vi "VAJ conti move.vi"(7 "move?":bool, 8 "error in (no error)":errorcluster, 9 "Position in":T1, 11 "move in":T3[](array[typedef])) -> (0 "error out":errorcluster, 1 "Position out":T1, 4 "Position out 2":T1)   [LabVIEW 2019]
uses:
  move cluster(VAJ).ctl
  move/position cluster.ctl
  <vilib>/Platform/TimedLoop/XDataNode/timing_clust.ctl
  <vilib>/Platform/TimedLoop/XDataNode/nitl_modes.ctl
  <vilib>/Platform/TimedLoop/XDataNode/wakeup.ctl
  <vilib>/platform/TimedLoop/XDataNode/XDataNode.xnode
  <vilib>/Platform/TimedLoop/XDataNode/XDNodeRunTimeDep.lvlib
panel:
  out "encoder array":dbl[](array[numeric])
  out "Waveform Chart":T2(graph)
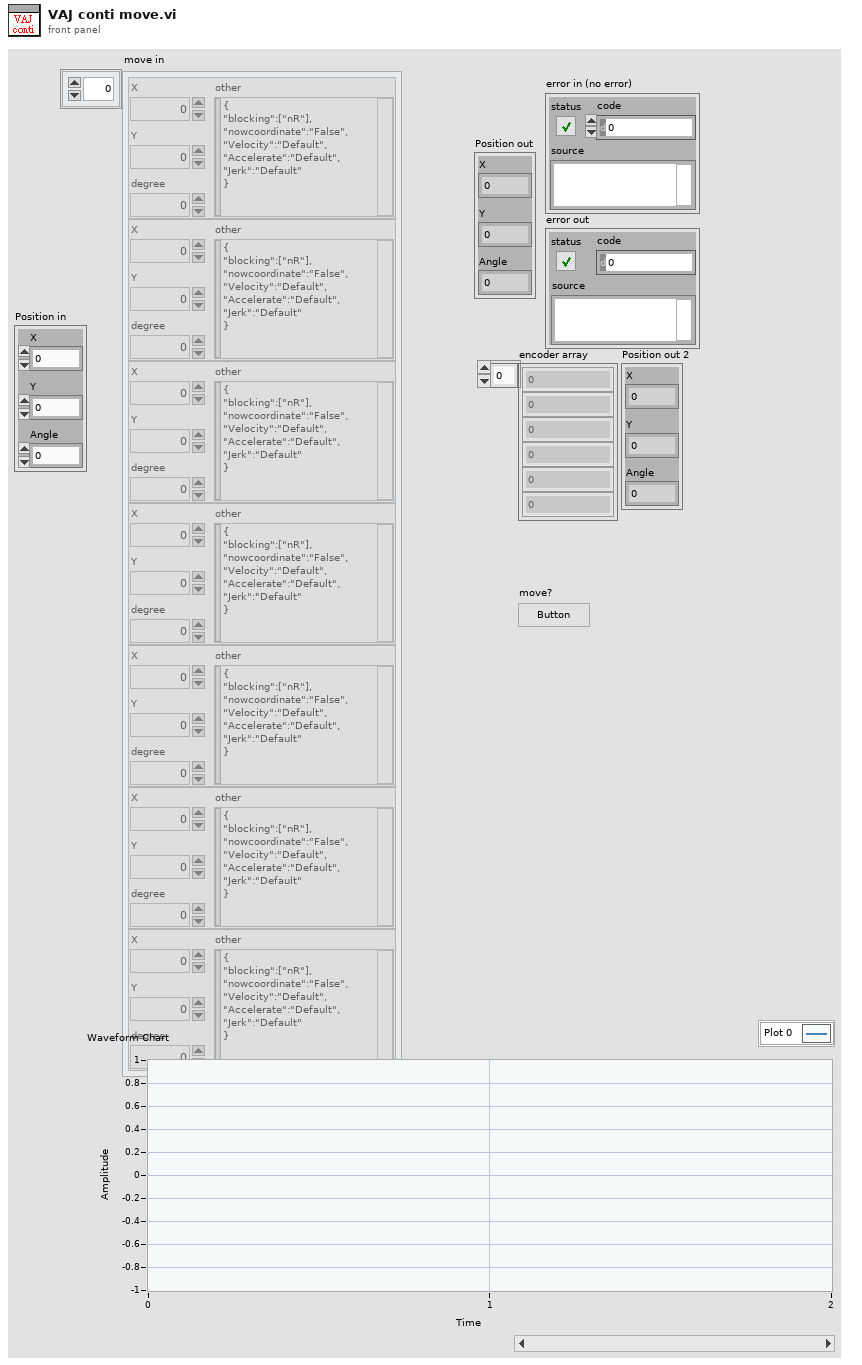
[diagram p1: front panel]
types:
  T1 = typedef "position cluster.ctl" = cluster{"X":dbl, "Y":dbl, "Angle":dbl}
  T2 = cluster{"[0]":dbl, "[1]":dbl, "[2]":dbl, "[3]":dbl, "[4]":dbl, "[5]":dbl, "[6]":dbl, "[7]":dbl, "[8]":dbl}
  T3 = typedef "move cluster(VAJ).ctl" = cluster{"X":dbl, "Y":dbl, "degree":dbl, "other":string}
  T4 = cluster{"Array":cluster{"Numeric":dbl, "Numeric":dbl}[], "direction out":dbl[], "rotate?":bool}[]
  T5 = typedef "BNO055 gyro 3axis.ctl" = cluster{"yaw":dbl, "pitch":dbl, "roll":dbl}
  T6 = typedef "XDNodeRunTimeDep.lvlib/timing_clust.ctl" = cluster{"Expected End [f-1]":u64, "Actual End [f-1]":u64, "Finished Late? [f-1]":bool, "Expected End [i-1]":u64, "Actual End [i-1]":u64, "Finished Late? [i-1]":bool, "Expected Start [i]":u64, "Actual Start [i]":u64, "Expected Start [f]":u64, "Actual Start [f]":u64, "Source Name":string, "Structure Name":string, "Period":i64, "Deadline":i64, "Offset":i64, "Start":i64, "Priority":i32, "Timeout":i32, "Mode":T7, "Wakeup Reason":T8, "Error":errorcluster, "Source Type":string, "Secondary Source Type":string, "Global End Time":u64, "Global Start Time":u64, "Frame Duration":u64, "Iteration Duration":u64, "Assigned CPU":i32, "I/O Scan Engine Mode":u32}
  T7 = typedef "XDNodeRunTimeDep.lvlib/nitl_modes.ctl" = enum32{"No Change", "Process missed periods, maintain original phase", "Discard missed periods, maintain original phase", "Process missed periods, ignore original phase", "Discard missed periods, ignore original phase"}
  T8 = typedef "XDNodeRunTimeDep.lvlib/wakeup.ctl" = enum32{"Normal", "Aborted", "Asynchronous wakeup", "Timing source error", "Timed loop error", "Timeout"}
  T9 = cluster{"Array":cluster{"Numeric":dbl, "Numeric":dbl}[], "direction out":dbl[], "rotate?":bool}
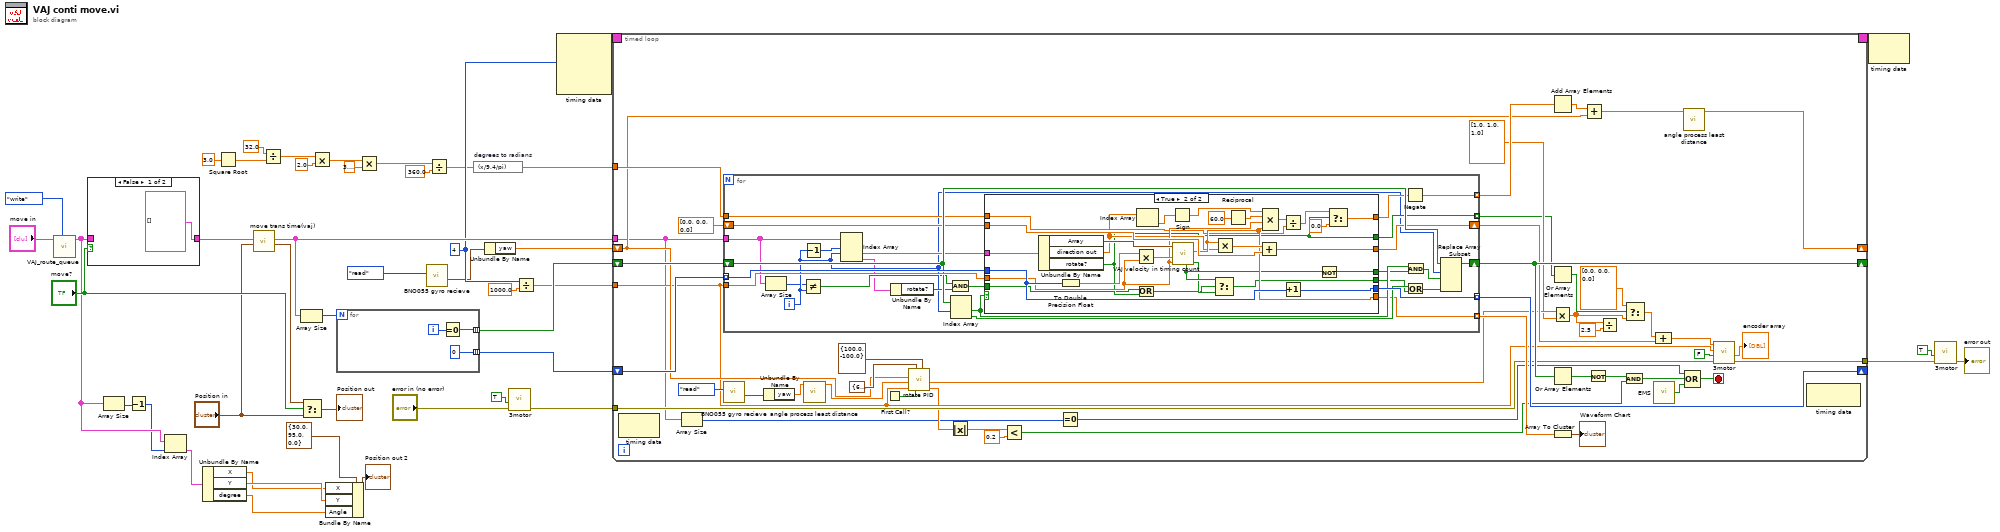
[diagram p0: block diagram]
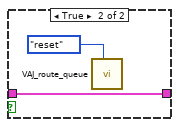
[diagram p2: hidden frame]
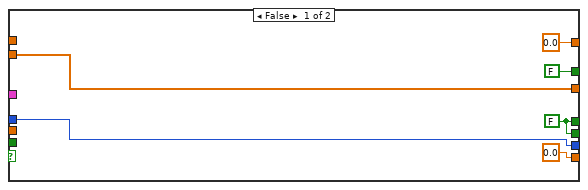
[diagram p3: hidden frame]
diagram:
  w39 = i64 4 ("Period")
  n1 = call "VAJ_route_queue.vi"("set"=enum16{"reset", "write"}."write", "move in"="move in") -> ("s? t:f"=w8:T3[])  [unwired: 9 in]
  n2 = case shown="False" "move?" {
    tunnel: [T3[] [] ("s? t:f") w48] -> w14
    tunnel: w8 -> [_ w48]
    frame False {
    }
    frame True {
      n3 = call "VAJ_route_queue.vi"("set"=enum16{"reset", "write"}."reset") -> ()  [unwired: 10 in, 1 out]
    }
  }
  n4 = Array Size(array=w8) -> (size(s)=w9:i32)
  n5 = Decrement(x=w9) -> (x-1=w7:i32)
  n6 = Index Array(array=w8, index=w7) -> (element=w6:T3)
  n7 = Unbundle By Name(w6) -> ("X"=w1:dbl, "Y"=w2:dbl, "degree"=w3:dbl)
  n8 = Square Root(x=3.0) -> (sqrt(x)=w23:dbl)
  n9 = call "move trans time(vaj)"("Position in"="Position in", "move in"=w14) -> ("Position out"=w11:T1, "speed create"=w43:T4)  [unwired: 8 in]
  n10 = Divide(x=32.0, y=w23) -> (x/y=w25:dbl)
  n11 = Array Size(array=w43) -> (size(s)=w42:i32)
  n12 = Select(t=w11, s="move?", f="Position in") -> (s? t:f=→"Position out":T1)
  n13 = Multiply(x=w25, y=2.0) -> (x*y=w28:dbl)
  n14 = Bundle By Name(cluster=T1 {"X"=30.0, "Y"=95.0, "Angle"=0.0} ("Position out 2"), "X"=w1, "Y"=w2, "Angle"=w3) -> (→"Position out 2":T1)
  n15 = for {
    N: w42 -> [_]
    tunnel: [w50] -> w41 mode=indexing
    tunnel: [0] -> w40 mode=indexing
    i -> [w49]
    n16 = Equal To 0?(x=w49) -> (x = 0?=w50:bool)
  }
  n17 = Multiply(x=w28, y=3.141592653589793) -> (x*y=w29:dbl)
  n18 = call "BNO055 gyro recieve.vi"("Enum"=enum16{"read", "write"}."read") -> ("read"=w20:T5)  [unwired: 10 in]
  n19 = Divide(x=w29, y=360.0) -> (x/y=w18:dbl)
  n20 = expression code="(x/9.4/pi)" "degrees to radians"(w18) -> (w17:dbl)
  n21 = Unbundle By Name(w20) -> ("yaw"=w19:dbl)
  n22 = call "3motor.vi"("error in (no error)"="error in (no error)", "Reset"=TRUE) -> ("error out"=w36:errorcluster)  [unwired: 8 in, 1 out]
  n23 = Divide(x=w39, y=1000.0) -> (x/y=w37:dbl)
  n24 = node-c288(w39) -> (w45:T6)  [unwired: 3 in]
  n25 = timed-loop {
    timing: w45 -> [_]
    timing-out: [_] -> w44
    tunnel: w43 -> [w59]
    shift-right: [w94] -> _
    shift-left: w41 -> [w98]
    shift-right: [w96] -> _
    shift-left: w40 -> [w97]
    tunnel: w37 -> [w73]
    tunnel: w36 -> [w87]
    tunnel: [w86] -> w32
    tunnel: w17 -> [w82]
    shift-right: [w79] -> _
    shift-left: w19 -> [w74]
    stop <- w85 stop-if-true
    n26 = node-c288() -> ()  [unwired: 1 in, 1 out]
    n27 = Array Size(array=w59) -> (size(s)=w58:i32)
    n28 = for {
      tunnel: w59 -> [w99]
      tunnel: w97 -> [w125] mode=indexing
      tunnel: [w124] -> w96 mode=indexing
      tunnel: w73 -> [w123]
      tunnel: [w115] -> w95 mode=indexing
      shift-right: [w114] -> w94
      shift-left: w98 -> [w122]
      shift-right: [w112] -> w89
      shift-left: dbl[] [0.0, 0.0, 0.0] -> [w113]
      tunnel: w82 -> [w111]
      tunnel: [w108] -> w81 mode=indexing
      tunnel: [w109] -> w64 mode=indexing
      i -> [w104]
      n29 = Array Size(array=w99) -> (size(s)=w100:i32)
      n30 = Not Equal?(x=w100, y=w104) -> (x != y?=w103:bool)
      n31 = Decrement(x=w104) -> (x-1=w106:i32)
      n32 = Index Array(array=w99, index #1=w106, index #2=w104) -> (element #2=w107:T9, element #3=w101:T9)  [unwired: 1 in, 1 out]
      n33 = Unbundle By Name(w101) -> ("rotate?"=w105:bool)
      n34 = And(x=w103, y=w105) -> (x .and. y?=w102:bool)
      n35 = Index Array(array=w122, index #1=w104) -> (element #1=w120:bool, element #2=w117:bool)  [unwired: 1 in]
      n36 = case shown="True" w120 {
        tunnel: w125 -> [w131 w157]
        tunnel: [w131 w159] -> w124
        tunnel: w123 -> [_ w148]
        tunnel: w107 -> [_ w156]
        tunnel: [w130 w153] -> w119
        tunnel: [w130 w134] -> w116
        tunnel: [0.0 ("velocity") w149] -> w115
        tunnel: [w128 w151] -> w112
        tunnel: w113 -> [w128 w150]
        tunnel: w111 -> [_ w146]
        tunnel: [0.0 ("f") w143] -> w110
        tunnel: [FALSE ("rotate?") w137] -> w109
        tunnel: w102 -> [_ w132]
        frame False {
          w130 = FALSE ("t4?")
        }
        frame True {
          n37 = Unbundle By Name(w156) -> ("Array"=w155:cluster{"Numeric":dbl, "Numeric":dbl}[], "direction out"=w140:dbl[], "rotate?"=w137:bool)
          n38 = To Double Precision Float(number=w157) -> (double precision float=w158:dbl)
          n39 = Multiply(x=w158, y=w148) -> (x*y=w154:dbl)
          n40 = Or(x=w132, y=w137) -> (x .or. y?=w133:bool)
          n41 = Index Array(array=w140) -> (element=w139:dbl)  [unwired: 1 in]
          n42 = Sign(1:w139) -> (0:w138:dbl)
          n43 = call "VAJ velocity in timing count.vi"("dt"=w148, "time"=w154, "Array"=w155) -> ("t4?"=w135:bool, "velocity"=w149:dbl, "finish"=w136:bool)  [unwired: 6 in]
          n44 = Select(t=w136, s=w133, f=w135) -> (s? t:f=w134:bool)
          n45 = Multiply(x=w149, y=w140) -> (x*y=w152:dbl[])
          n46 = Reciprocal(x=60.0) -> (1/x=w142:dbl)
          n47 = Add(x=w152, y=w150) -> (x+y=w151:dbl[])
          n48 = Compound Arithmetic op=MULTIPLY(w138, w142, w148, w149) -> (w147:dbl)
          n49 = Divide(x=w147, y=w146) -> (x/y=w145:dbl)
          n50 = Increment(x=w157) -> (x+1=w159:i32)
          n51 = Not(x=w136) -> (.not. x?=w153:bool)
          n52 = Select(t=w145, s=w137, f=0.0) -> (s? t:f=w143:dbl)
        }
      }
      n53 = Negate(x=w110) -> (-x=w108:dbl)
      n54 = Or(x=w117, y=w116) -> (x .or. y?=w118:bool)
      n55 = And(x=w120, y=w119) -> (x .and. y?=w121:bool)
      n56 = Replace Array Subset(array=w122, new element #1=w121, index #1=w104, new element #2=w118) -> (w114:bool[])  [unwired: 1 in]
    }
    n57 = call "BNO055 gyro recieve.vi"("Enum"=enum16{"read", "write"}."read") -> ("read"=w77:T5)  [unwired: 10 in]
    n58 = Unbundle By Name(w77) -> ("yaw"=w54:dbl)
    n59 = call "angle process least distance.vi"("Numeric in"=w54) -> ("Numeric out"=w53:dbl)  [unwired: 10 in]
    n60 = First Call?() -> (First Call?: T/F=w56:bool)
    n61 = call "rotate PID.vi"("output range"=cluster{"output high":dbl, "output low":dbl} {"output high"=100.0, "output low"=-100.0}, "s"=w56, "PID"=cluster{"Kp":dbl, "Ki":dbl, "Kd":dbl} {"Kp"=6.0, "Ki"=0.0, "Kd"=0.0005}, "dt (s)"=w73, "Processer"=w53, "setpoint"=w74) -> ("e(t)"=w72:dbl, "out"=w67:dbl)  [unwired: 4 in]
    n62 = Absolute Value(x=w72) -> (abs(x)=w71:dbl)
    n63 = Less?(x=w71, y=0.2) -> (x < y?=w68:bool)
    n64 = Equal To 0?(x=w58) -> (x = 0?=w57:bool)
    n65 = Add Array Elements(numeric array=w81) -> (sum=w52:dbl)
    n66 = Or Array Elements(Boolean array=w64) -> (logical OR=w62:bool)
    n67 = Multiply(x=w67, y=dbl[] [1.0, 1.0, 1.0]) -> (x*y=w61:dbl[])
    n68 = Or Array Elements(Boolean array=w94) -> (logical OR=w93:bool)
    n69 = Array To Cluster(array=w95) -> (cluster=→"Waveform Chart":T2)
    n70 = Add(x=w52, y=w74) -> (x+y=w80:dbl)
    n71 = Not(x=w93) -> (.not. x?=w92:bool)
    n72 = Divide(x=w61, y=2.5) -> ()  [unwired: 1 out]
    n73 = And(x=w92, y=w68) -> (x .and. y?=w69:bool)
    n74 = Select(t=dbl[] [0.0, 0.0, 0.0], s=w62, f=w61) -> (s? t:f=w63:dbl[])
    n75 = call "EMS.vi"() -> ("A/DIO4 (Pin 19)"=w84:bool)
    n76 = Compound Arithmetic op=ADD(w63, w89) -> (w65:dbl[])
    n77 = call "angle process least distance.vi"("Numeric in"=w80) -> ("Numeric out"=w79:dbl)  [unwired: 10 in]
    n78 = Compound Arithmetic op=OR(w57, w69, w84) -> (w85:bool)
    n79 = call "3motor.vi"("error in (no error)"=w87, "Reset"=FALSE, "dt(s)"=w73, "Motor speed"=w65) -> ("error out"=w86:errorcluster, "encoder array"=→"encoder array":dbl[])  [unwired: 6 in]
    n80 = node-c288() -> ()  [unwired: 1 in, 1 out]
  }
  n81 = node-c288(w44) -> ()  [unwired: 1 out]
  n82 = call "3motor.vi"("error in (no error)"=w32, "Reset"=TRUE) -> ("error out"=→"error out":errorcluster)  [unwired: 8 in, 1 out]
